vi "CCD3000 Jacobian Transformation v10.4.0.vi"(3 "Spectrum-Array In":dbl[][](array[numeric])) -> (0 "Spectrum-Array Out":dbl[][](array[numeric]), 1 "Spectrum-Cluster":T1(array[cluster]))   [LabVIEW 2010]
uses:
  <vilib>/Analysis/NI_AALBase.lvlib
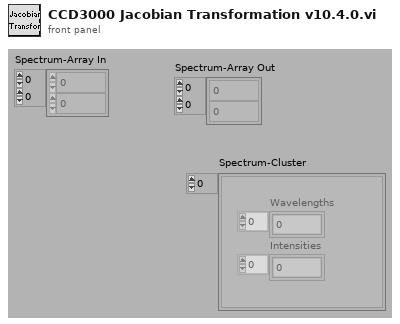
[diagram p1: front panel]
types:
  T1 = cluster{"Intensities":dbl[], "Wavelengths":dbl[]}[]
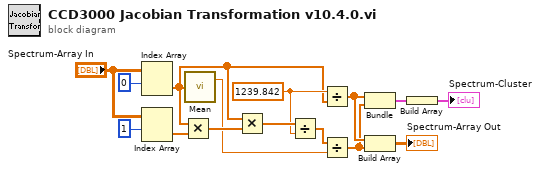
[diagram p0: block diagram]
diagram:
  w7 = 1239.842 ("x")
  n1 = Index Array(array="Spectrum-Array In", index (row)=0 ("disabled index (col)")) -> (element=w5:dbl[])  [unwired: 1 in]
  n2 = Index Array(array="Spectrum-Array In", index (row)=1 ("disabled index (col)")) -> (element=w10:dbl[])  [unwired: 1 in]
  n3 = Multiply(x=w5, y=w10) -> (x*y=w9:dbl[])
  n4 = call <vilib>:"Mean.vi"("X"=w5) -> ("mean"=w6:dbl)  [unwired: 1 out]
  n5 = Multiply(x=w5, y=w9) -> (x*y=w8:dbl[])
  n6 = Divide(x=w8, y=w7) -> (x/y=w4:dbl[])
  n7 = Divide(x=w7, y=w5) -> (x/y=w11:dbl[])
  n8 = Divide(x=w4, y=w6) -> (x/y=w3:dbl[])
  n9 = Bundle(w11, w3) -> (w14:cluster{dbl[], dbl[]})  [unwired: 1 in]
  n10 = Build Array(w11, w3) -> (→"Spectrum-Array Out":dbl[][])
  n11 = Build Array(w14) -> (→"Spectrum-Cluster":cluster{dbl[], dbl[]}[])
